vi "Autonomous Independent.vi"   [LabVIEW 2017]
doc: "This VI is called when autonomous begins, and will automatically be terminated when autonomous ends. You can carry out timed or sensor driven robot movement independently without needing to return to the caller."
uses:
  <vilib>/Rock Robotics/WPI/Ultrasonic/WPI_UltrasonicRangeUnits.ctl
  <vilib>/Rock Robotics/WPI/ThirdParty/Sensors/navX/_TypeDefs/FRIC_navX_DeviceNumbersTypeDef.ctl
  <vilib>/Rock Robotics/WPI/Utilities/WPI_GetSetVariantRefNum.vi
  <vilib>/Rock Robotics/Network Tables/NT Read String.vi
  Robot Global Data.vi
  <vilib>/Rock Robotics/WPI/RobotDrive/WPI_RobotDriveArcadeDrive_Standard(NoSaturation).vi
  <vilib>/Rock Robotics/WPI/Ultrasonic/WPI_SonarSRF04DigitalRefNum Registry Get.vi
  <vilib>/Rock Robotics/WPI/Ultrasonic/WPI_SonarSRF04DigitalGetRange.vi
  <vilib>/Rock Robotics/Network Tables/NT Write Numeric Array.vi
panel:
  # "Be sure to right-click and choose Data Operations>>Make Current Value default if you want to save the array values with the VI"
types:
  T1 = typedef "WPI_JoystickDevRef.ctl" = cluster{"Device":T2}
  T2 = typedef "WPI_JoystickDeviceEnum.ctl" = enum16{"USB 0", "USB 1", "USB 2", "USB 3", "USB 4", "USB 5"}
  T3 = typedef "WPI_UltrasonicRangeUnits.ctl" = enum16{"inches", "mm"}
  T4 = typedef "FRIC_navX_DeviceNumbersTypeDef.ctl" = enum16{"Dev0", "Dev1", "Dev2", "Dev3"}
  T5 = typedef "WPI_RobotDriveDevRef.ctl" = cluster{"DevStatus":errorcluster, "Motors[]":T6[], "Square Inputs":bool, "Max Output":dbl}
  T6 = typedef "WPI_MotorControlDeviceRef.ctl" = cluster{"DeviceStatus":errorcluster, "Type":T7, "PWM":cluster{"PWM Channel":T8, "DeadBand":T9}, "CAN":cluster{"Device Number":u8, "SetOutput VI Ref":variant, "GetOutput VI Ref":variant, "Enable VI Ref":variant, "Disable VI Ref":variant, "Data":variant}, "Invert":bool, "DIO PWM":cluster{"PWM \"Enable\" Channel":T8, "DIOChannel":T10, "PWM Rate":dbl}}
  T7 = typedef "WPI_MotorControlType.ctl" = enum16{"PWM", "CAN", "DIO PWM"}
  T8 = typedef "FPGA_DIOPWMChannel.ctl" = enum8{"PWM 0", "PWM 1", "PWM 2", "PWM 3", "PWM 4", "PWM 5", "PWM 6", "PWM 7", "PWM 8", "PWM 9", "PWM MXP 0", "PWM MXP 1", "PWM MXP 2", "PWM MXP 3", "PWM MXP 4", "PWM MXP 5", "PWM MXP 6", "PWM MXP 7", "PWM MXP 8", "PWM MXP 9", "Invalid"}
  T9 = typedef "WPI_PWMDeadband.ctl" = cluster{"Name":string, "maxPositivePwm":i32, "minPositivePwm":i32, "centerPwm":i32, "maxNegativePwm":i32, "minNegativePwm":i32, "angularRange":u16}
  T10 = typedef "FPGA_DIOChannel.ctl" = enum8{"DIO 0", "DIO 1", "DIO 2", "DIO 3", "DIO 4", "DIO 5", "DIO 6", "DIO 7", "DIO 8", "DIO 9", "DIO MXP 0", "DIO MXP 1", "DIO MXP 2", "DIO MXP 3", "DIO MXP 4", "DIO MXP 5", "DIO MXP 6", "DIO MXP 7", "DIO MXP 8", "DIO MXP 9", "DIO MXP 10", "DIO MXP 11", "DIO MXP 12", "DIO MXP 13", "DIO MXP 14", "DIO MXP 15", "SPI Port CS1", "SPI Port CS2", "SPI Port CS3", "SPI Port MISO", "SPI Port MOSI", "Invalid"}
  T11 = cluster{"Type":enum16{"Normal Object", "Color Object"}, "Signature":u16, "X":u16, "Y":u16, "Width":u16, "Height":u16, "Angle":u16}[]
  T12 = cluster{"Type":enum16{"Normal Object", "Color Object"}, "Signature":u16, "X":u16, "Y":u16, "Width":u16, "Height":u16, "Angle":u16}
  T13 = typedef "WPI_UltrasonicDeviceRef.ctl" = cluster{"DevStatus":errorcluster, "Ping Channel":T10, "Echo Channel":T10, "CntIndex":T14}
  T14 = typedef "FPGA_CounterCtrSystemIndex.ctl" = enum8{"Ctr 0", "Ctr 1", "Ctr 2", "Ctr 3", "Ctr 4", "Ctr 5", "Ctr 6", "Ctr 7", "Invalid"}
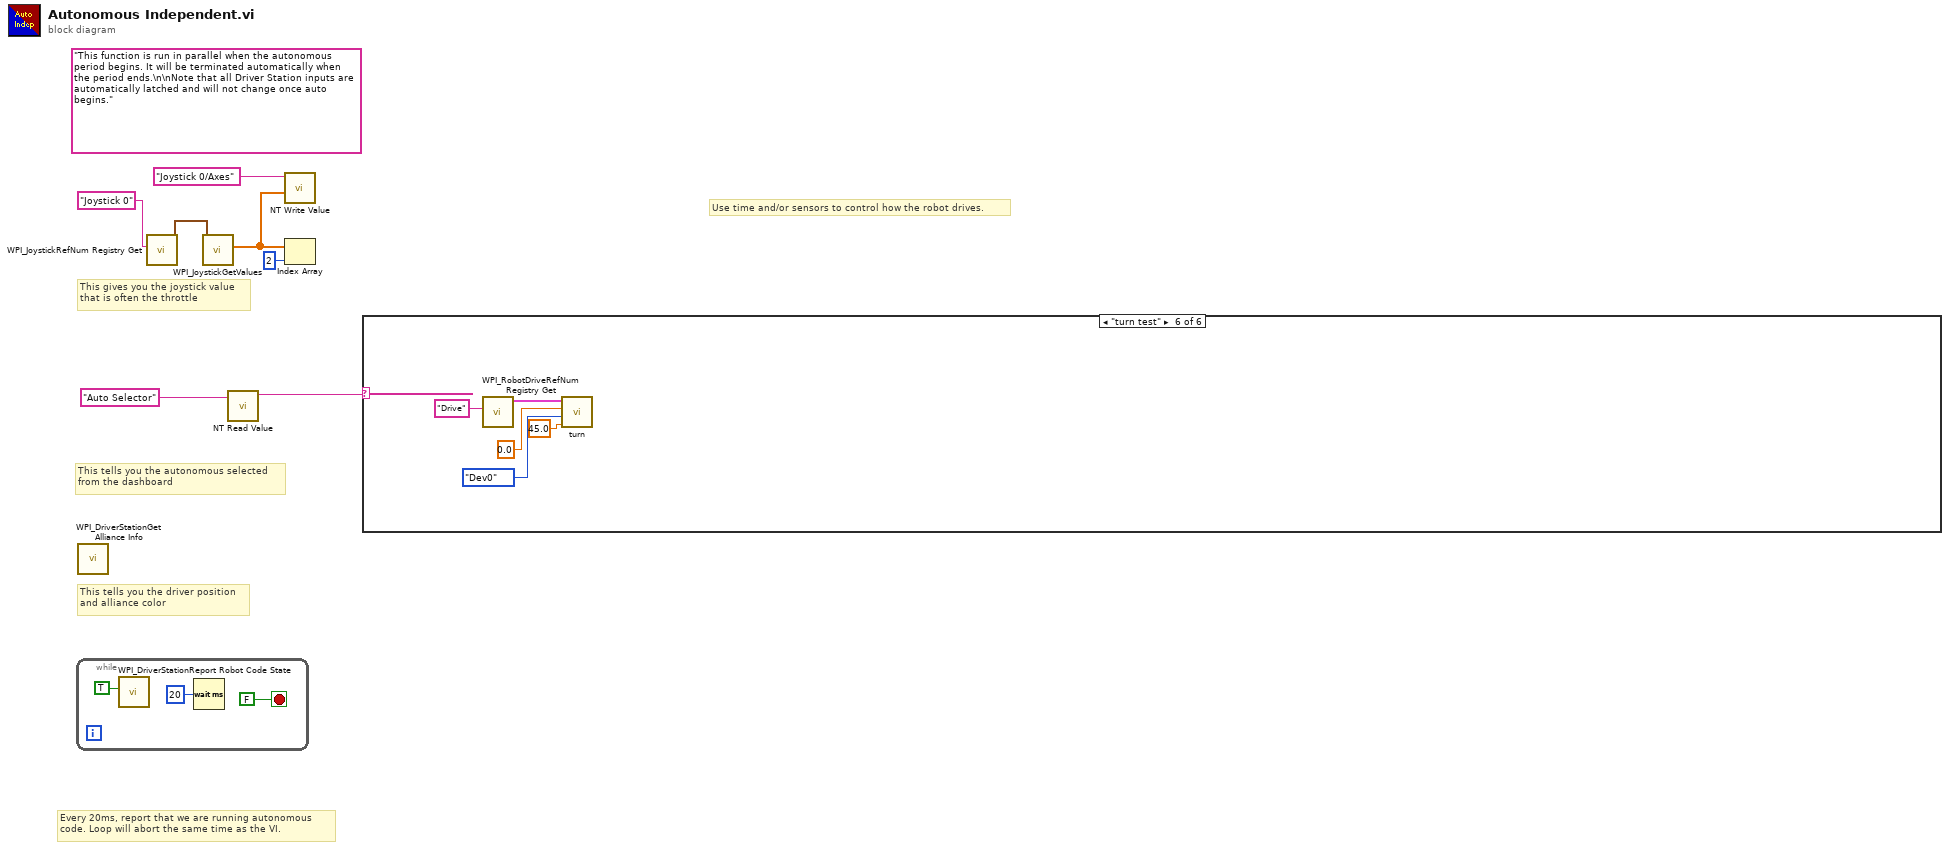
[diagram p0: block diagram]
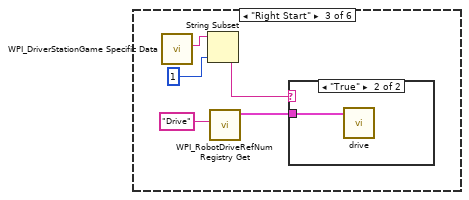
[diagram p4: hidden frame]
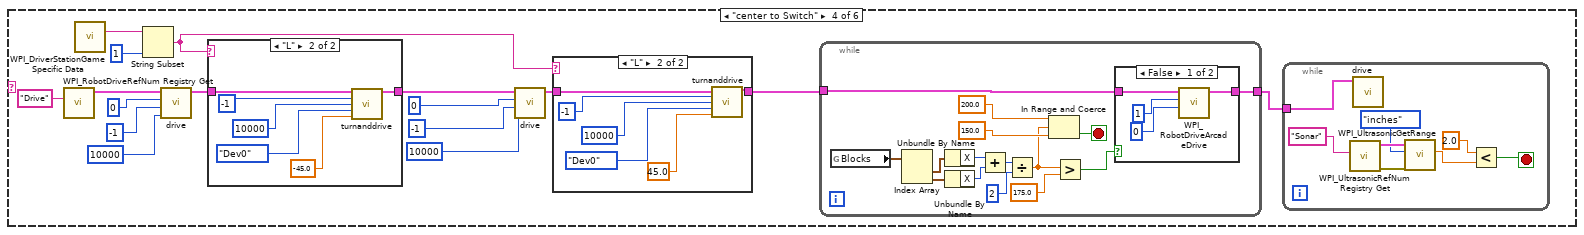
[diagram p6: hidden frame]
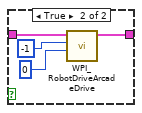
[diagram p7: hidden frame]
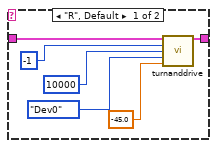
[diagram p8: hidden frame]
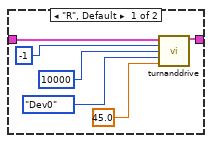
[diagram p9: hidden frame]
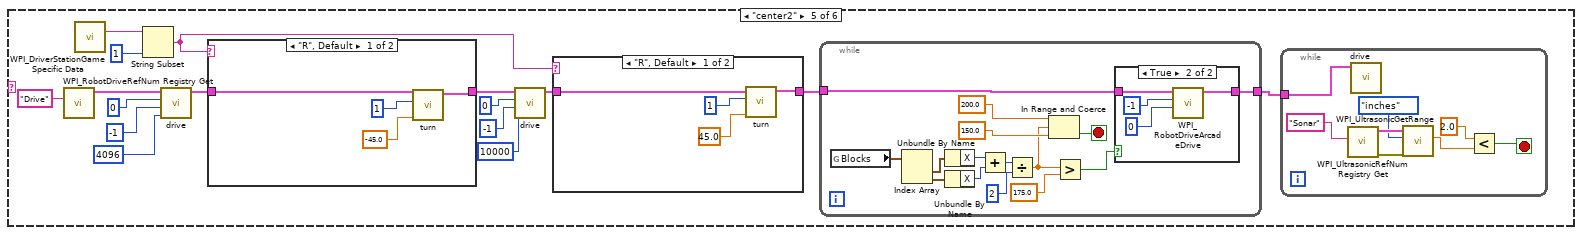
[diagram p10: hidden frame]
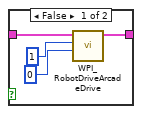
[diagram p11: hidden frame]
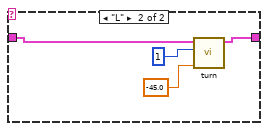
[diagram p12: hidden frame]
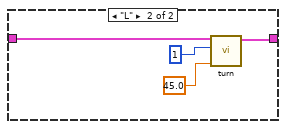
[diagram p13: hidden frame]
diagram:
  (unwired) "This function is run in parallel when the autonomous period begins. It will be terminated automatically when the period ends.\n\nNote that all Driver Station inputs are automatically latched and will not change once auto begins."
  # "This tells you the autonomous selected\nfrom the dashboard"
  # "Every 20ms, report that we are running autonomous\ncode. Loop will abort the same time as the VI."
  # "This gives you the joystick value\nthat is often the throttle"
  # "Use time and/or sensors to control how the robot drives."
  # "This tells you the driver position\nand alliance color"
  n1 = while {
    stop <- FALSE stop-if-true
    n2 = call <vilib>:"WPI_DriverStationReport Robot Code State.vi"("Autonomous"=TRUE) -> ()  [unwired: 10 in, 1 out]
    n3 = Wait (ms)(milliseconds to wait=u32 20) -> ()  [unwired: 1 out]
  }
  n4 = call <vilib>:"WPI_DriverStationGet Alliance Info.vi"() -> ()  [unwired: 12 out]
  n5 = call <vilib>:"WPI_JoystickRefNum Registry Get.vi"("refnum name"="Joystick 0") -> ("JoystickDevRef"=w6:T1)  [unwired: 1 in, 9 out]
  n6 = call <vilib>:"WPI_JoystickGetValues.vi"("JoystickDevRef"=w6) -> ("Axes"=w2:dbl[])  [unwired: 6 in, 4 out]
  n7 = call-poly <vilib>:"NT Read Value.vi"("Name"="Auto Selector") -> ("String"=w3:string)  [unwired: 9 in, 1 out]
  n8 = call-poly <vilib>:"NT Write Value.vi"("Numeric Array"=w2, "Name"="Joystick 0/Axes") -> ()  [unwired: 9 in, 1 out]
  n9 = Index Array(array=w2, index=2) -> ()  [unwired: 1 out]
  n10 = case shown="\"turn test\"" w3 {
    frame Default {
    }
    frame "Alternative 1" {
    }
    frame "Right Start" {
      n11 = call <vilib>:"WPI_DriverStationGame Specific Data.vi"() -> ("Game Specific Data"=w15:string)  [unwired: 11 in]
      n12 = String Subset(string=w15, length (rest)=1 ("length (rest)")) -> (substring=w12:string)  [unwired: 1 in]
      n13 = call <vilib>:"WPI_RobotDriveRefNum Registry Get.vi"("refnum name"="Drive") -> ("RobotDriveDevRef"=w13:T5)  [unwired: 9 in, 1 out]
      n14 = case shown="\"True\"" w12 {
        tunnel: w13 -> [_ w16]
        frame "False", Default {
        }
        frame "True" {
          n15 = call "drive.vi"("RobotDriveDevRef"=w16) -> ()  [unwired: 10 in, 1 out]
        }
      }
    }
    frame "center to Switch" {
      n16 = call <vilib>:"WPI_RobotDriveRefNum Registry Get.vi"("refnum name"="Drive") -> ("RobotDriveDevRef"=w26:T5)  [unwired: 9 in, 1 out]
      n17 = call <vilib>:"WPI_DriverStationGame Specific Data.vi"() -> ("Game Specific Data"=w30:string)  [unwired: 11 in]
      n18 = String Subset(string=w30, length (rest)=1 ("length (rest)")) -> (substring=w28:string)  [unwired: 1 in]
      n19 = call "drive.vi"("distance"=10000, "Y"=-1, "X"=0, "RobotDriveDevRef"=w26) -> ("RobotDriveDevRef dup."=w27:T5)  [unwired: 7 in]
      n20 = case shown="\"L\"" w28 {
        tunnel: w27 -> [w78 w87]
        tunnel: [w77 w86] -> w23
        frame "R", Default {
          n21 = call "turnanddrive.vi"("RobotDriveDevRef"=w78, "y"=-1, "distance"=10000, "Device Number"=FRIC_navX_DeviceNumbersTypeDef."Dev0", "Angle"=45.0 ("Angel")) -> ("RobotDriveDevRef dup."=w77:T5)  [unwired: 10 in]
        }
        frame "L" {
          n22 = call "turnanddrive.vi"("RobotDriveDevRef"=w87, "y"=-1, "distance"=10000, "Device Number"=FRIC_navX_DeviceNumbersTypeDef."Dev0", "Angle"=-45.0 ("Angel")) -> ("RobotDriveDevRef dup."=w86:T5)  [unwired: 10 in]
        }
      }
      n23 = call "drive.vi"("distance"=10000, "Y"=-1, "X"=0, "RobotDriveDevRef"=w23) -> ("RobotDriveDevRef dup."=w22:T5)  [unwired: 7 in]
      n24 = case shown="\"L\"" w28 {
        tunnel: w22 -> [w65 w73]
        tunnel: [w64 w72] -> w29
        frame "R", Default {
          n25 = call "turnanddrive.vi"("RobotDriveDevRef"=w65, "y"=-1, "distance"=10000, "Device Number"=FRIC_navX_DeviceNumbersTypeDef."Dev0", "Angle"=-45.0 ("Angel")) -> ("RobotDriveDevRef dup."=w64:T5)  [unwired: 10 in]
        }
        frame "L" {
          n26 = call "turnanddrive.vi"("RobotDriveDevRef"=w73, "y"=-1, "distance"=10000, "Device Number"=FRIC_navX_DeviceNumbersTypeDef."Dev0", "Angle"=45.0 ("Angel")) -> ("RobotDriveDevRef dup."=w72:T5)  [unwired: 10 in]
        }
      }
      n27 = while {
        tunnel: w29 -> [w41]
        tunnel: [w42] -> w17
        stop <- w48 stop-if-true
        n28 = global read "Robot Global Data.vi" "Blocks"() -> (w55:T11)
        n29 = Index Array(array=w55) -> (element #1=w54:T12, element #2=w53:T12)  [unwired: 2 in]
        n30 = Unbundle By Name(w54) -> ("X"=w52:u16)
        n31 = Unbundle By Name(w53) -> ("X"=w51:u16)
        n32 = Add(x=w52, y=w51) -> (x+y=w50:u16)
        n33 = Divide(x=w50, y=u16 2) -> (x/y=w47:dbl)
        n34 = In Range and Coerce(upper limit=200.0, x=w47, lower limit=150.0) -> (In Range?=w48:bool)  [unwired: 1 out]
        n35 = Greater?(x=w47, y=175.0) -> (0:w45:bool)
        n36 = case shown="False" w45 {
          tunnel: w41 -> [w59 w61]
          tunnel: [w56 w60] -> w42
          frame False {
            n37 = call-poly <vilib>:"WPI_RobotDriveArcadeDrive.vi"("Y axis value"=0, "X axis value"=1, "RobotDriveDevRef"=w59) -> ("RobotDriveDevRef"=w56:T5)  [unwired: 6 in, 2 out]
          }
          frame True {
            n38 = call-poly <vilib>:"WPI_RobotDriveArcadeDrive.vi"("Y axis value"=0, "X axis value"=-1, "RobotDriveDevRef"=w61) -> ("RobotDriveDevRef"=w60:T5)  [unwired: 6 in, 2 out]
          }
        }
      }
      n39 = while {
        tunnel: w17 -> [w40]
        stop <- w34 stop-if-true
        n40 = call-poly <vilib>:"WPI_UltrasonicRefNum Registry Get.vi"("refnum name"="Sonar") -> ("error out"=w38:errorcluster, "SonarSRF04DevRef"=w39:T13)  [unwired: 9 in]
        n41 = call "drive.vi"("RobotDriveDevRef"=w40) -> ()  [unwired: 10 in, 1 out]
        n42 = call-poly <vilib>:"WPI_UltrasonicGetRange.vi"("error in (no error)"=w38, "ping time (s)"=WPI_UltrasonicRangeUnits."inches" ("Range Units"), "SonarSRF04DevRef"=w39) -> ("Distance"=w36:dbl)  [unwired: 6 in, 2 out]
        n43 = Less?(x=2.0, y=w36) -> (x < y?=w34:bool)
      }
    }
    frame "center2" {
      n44 = call <vilib>:"WPI_RobotDriveRefNum Registry Get.vi"("refnum name"="Drive") -> ("RobotDriveDevRef"=w97:T5)  [unwired: 9 in, 1 out]
      n45 = call <vilib>:"WPI_DriverStationGame Specific Data.vi"() -> ("Game Specific Data"=w101:string)  [unwired: 11 in]
      n46 = String Subset(string=w101, length (rest)=1 ("length (rest)")) -> (substring=w99:string)  [unwired: 1 in]
      n47 = call "drive.vi"("distance"=4096, "Y"=-1, "X"=0, "RobotDriveDevRef"=w97) -> ("RobotDriveDevRef dup."=w98:T5)  [unwired: 7 in]
      n48 = case shown="\"R\", Default" w99 {
        tunnel: w98 -> [w143 w148]
        tunnel: [w144 w150] -> w94
        frame "R", Default {
          n49 = call "turn.vi"("Angle"=-45.0, "y"=1, "RobotDriveDevRef"=w143) -> ("RobotDriveDevRef dup."=w144:T5)  [unwired: 8 in]
        }
        frame "L" {
          n50 = call "turn.vi"("Angle"=45.0, "y"=1, "RobotDriveDevRef"=w148) -> ("RobotDriveDevRef dup."=w150:T5)  [unwired: 8 in]
        }
      }
      n51 = call "drive.vi"("distance"=10000, "Y"=-1, "X"=0, "RobotDriveDevRef"=w94) -> ("RobotDriveDevRef dup."=w93:T5)  [unwired: 7 in]
      n52 = case shown="\"R\", Default" w99 {
        tunnel: w93 -> [w136 w139]
        tunnel: [w135 w140] -> w100
        frame "R", Default {
          n53 = call "turn.vi"("Angle"=45.0, "y"=1, "RobotDriveDevRef"=w136) -> ("RobotDriveDevRef dup."=w135:T5)  [unwired: 8 in]
        }
        frame "L" {
          n54 = call "turn.vi"("Angle"=-45.0, "y"=1, "RobotDriveDevRef"=w139) -> ("RobotDriveDevRef dup."=w140:T5)  [unwired: 8 in]
        }
      }
      n55 = while {
        tunnel: w100 -> [w112]
        tunnel: [w113] -> w88
        stop <- w119 stop-if-true
        n56 = global read "Robot Global Data.vi" "Blocks"() -> (w126:T11)
        n57 = Index Array(array=w126) -> (element #1=w125:T12, element #2=w124:T12)  [unwired: 2 in]
        n58 = Unbundle By Name(w125) -> ("X"=w123:u16)
        n59 = Unbundle By Name(w124) -> ("X"=w122:u16)
        n60 = Add(x=w123, y=w122) -> (x+y=w121:u16)
        n61 = Divide(x=w121, y=u16 2) -> (x/y=w118:dbl)
        n62 = In Range and Coerce(upper limit=200.0, x=w118, lower limit=150.0) -> (In Range?=w119:bool)  [unwired: 1 out]
        n63 = Greater?(x=w118, y=175.0) -> (0:w116:bool)
        n64 = case shown="True" w116 {
          tunnel: w112 -> [w130 w132]
          tunnel: [w127 w131] -> w113
          frame False {
            n65 = call-poly <vilib>:"WPI_RobotDriveArcadeDrive.vi"("Y axis value"=0, "X axis value"=1, "RobotDriveDevRef"=w130) -> ("RobotDriveDevRef"=w127:T5)  [unwired: 6 in, 2 out]
          }
          frame True {
            n66 = call-poly <vilib>:"WPI_RobotDriveArcadeDrive.vi"("Y axis value"=0, "X axis value"=-1, "RobotDriveDevRef"=w132) -> ("RobotDriveDevRef"=w131:T5)  [unwired: 6 in, 2 out]
          }
        }
      }
      n67 = while {
        tunnel: w88 -> [w111]
        stop <- w105 stop-if-true
        n68 = call-poly <vilib>:"WPI_UltrasonicRefNum Registry Get.vi"("refnum name"="Sonar") -> ("error out"=w109:errorcluster, "SonarSRF04DevRef"=w110:T13)  [unwired: 9 in]
        n69 = call "drive.vi"("RobotDriveDevRef"=w111) -> ()  [unwired: 10 in, 1 out]
        n70 = call-poly <vilib>:"WPI_UltrasonicGetRange.vi"("error in (no error)"=w109, "ping time (s)"=WPI_UltrasonicRangeUnits."inches" ("Range Units"), "SonarSRF04DevRef"=w110) -> ("Distance"=w107:dbl)  [unwired: 6 in, 2 out]
        n71 = Less?(x=2.0, y=w107) -> (x < y?=w105:bool)
      }
    }
    frame "turn test" {
      n72 = call <vilib>:"WPI_RobotDriveRefNum Registry Get.vi"("refnum name"="Drive") -> ("RobotDriveDevRef"=w151:T5)  [unwired: 9 in, 1 out]
      n73 = call "turn.vi"("Angle"=45.0, "Device Number"=FRIC_navX_DeviceNumbersTypeDef."Dev0", "y"=0.0 ("Y axis value"), "RobotDriveDevRef"=w151) -> ()  [unwired: 7 in, 1 out]
    }
  }
